vi "IPI_Cal_Step3_Bottom.vi"(8 "error in":errorcluster, 10 "Image In":T1, 11 "Session In":T2) -> (0 "error out":errorcluster, 2 "mm":sgl, 3 "Image":T1(plugin-control))   [LabVIEW 2015]
uses:
  <vilib>/userdefined/High Color/IMAQdx.ctl
  <vilib>/vision/Image Controls.llb/IMAQ Image.ctl
  <vilib>/vision/driver/NI_Vision_Acquisition_Software.lvlib
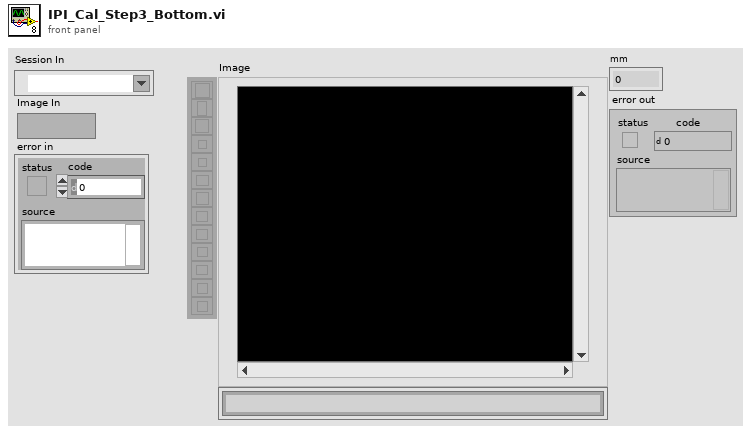
[diagram p1: front panel]
types:
  T1 = typedef "IMAQ Image.ctl" = refnum<image>
  T2 = typedef "IMAQdx.ctl" = refnum<k21>
  T3 = cluster{"Global Rectangle":i32[], "Contours":cluster{"ID":enum32{"External", "Internal"}, "Type":u32, "Coordinates":i32[]}[]}
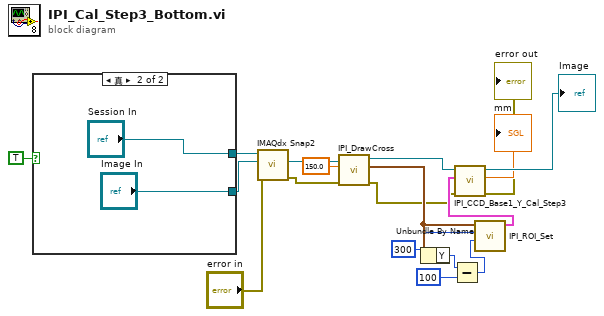
[diagram p0: block diagram]
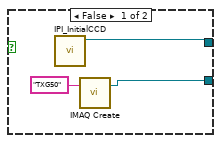
[diagram p2: hidden frame]
diagram:
  n1 = case shown="真" TRUE {
    tunnel: [w21 "Session In"] -> w12
    tunnel: [w19 "Image In"] -> w11
    frame False {
      n2 = call "IPI_InitialCCD.vi"() -> ("Session Out"=w21:T2)  [unwired: 10 in, 1 out]
      n3 = call "IMAQ Create"("Image Name"="TXG50") -> ("New Image"=w19:T1)  [unwired: 4 in, 1 out]
    }
    frame True {
    }
  }
  n4 = call <vilib>:"IMAQdx Snap2.vi"("error in"="error in", "Image In"=w11, "Session In"=w12) -> ("error out"=w3:errorcluster, "Image Out"=w18:T1)  [unwired: 6 in, 1 out]
  n5 = call "IPI_DrawCross.vi"("error in (no error)"=w3, "X"=150.0 ("R"), "Image In"=w18) -> ("error out"=w2:errorcluster, "XYCenter"=w14:cluster{"X":i32, "Y":i32}, "Image Out"=w16:T1)  [unwired: 6 in]
  n6 = Unbundle By Name(w14) -> ("Y"=w7:i32)
  n7 = Subtract(x=w7, y=100) -> (x-y=w5:i32)
  n8 = call "IPI_ROI_Set.vi"("Y"=w5, "X"=300 ("y"), "XYCenter"=w14) -> ("ROI"=w15:T3)  [unwired: 8 in]
  n9 = call "IPI_CCD_Base1_Y_Cal_Step3.vi"("error in"=w2, "ROI Descriptor (Find Straight Edge 1)"=w15, "Image In"=w16) -> ("error out"=→"error out":errorcluster, "mm"=→"mm":sgl, "Image"=→"Image":T1)  [unwired: 6 in]
